vi "GetGaussianKernel.vi"(8 "error in":errorcluster, 10 "Sigma":dbl=-1.0, 11 "kSize":i32=3 step=2) -> (0 "error out":errorcluster, 3 "Kernel":dbl[](array[numeric]))   [LabVIEW 2020, in "OpenLvVision_OpenCv.lvlib"]
doc: "Returns Gaussian filter coefficients."
uses:
  OpenLvVision_OpenCv.lvlib
  Dlls/OlvOpenCvWrapper.dll
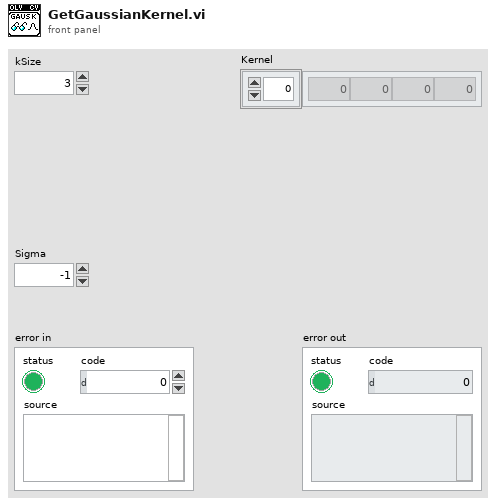
[diagram p1: front panel]
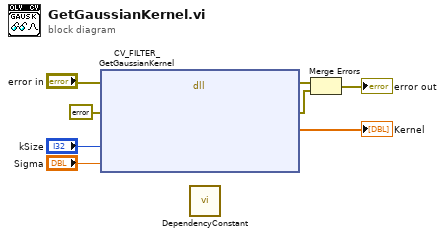
[diagram p0: block diagram]
diagram:
  n1 = dll-call lib="C:/Users/lukas/Downloads/OpenLvVision_OpenCv/SourceCode/LabView/OpenLvVision_OpenCv/Dlls/OlvOpenCvWrapper.dll" fn="CV_FILTER_GetGaussianKernel"(error in="error in", "Error"=errorcluster {"status"=FALSE, "code"=0, "source"=""} ("error constant"), "kSize"="kSize", "sigma"="Sigma") -> (error out=w7:errorcluster, "Error"=w6:errorcluster, "dst"=→"Kernel":dbl[])  [unwired: 6 in, 1 out]
  n2 = call "DependencyConstant.vi"() -> ()  [unwired: 12 in]
  n3 = Merge Errors(w7, w6) -> (→"error out":errorcluster)
